vi "main.vi"() -> ()   [LabVIEW 2023]
uses:
  Laser_Ethernet_class/Laser_Ethernet.lvclass
  Laser Ethernet Rack_class/Laser Ethernet Rack.lvclass
  Laser Ethernet Cabinet_class/Laser Ethernet Cabinet.lvclass
  C:/Users/TimBerrier/Code/LabVIEW/Source/APIs/IPG/ipg_tcp/Laser_Ethernet_class/Laser_Ethernet.lvclass
panel:
  in  "Rack?":bool
  in  "address 2":string
  in  "timeout (ms) 2":i32=5000
  in  "remote port or service name 2":u16=5100
  out "Connected 2":bool
  out "error out 2":errorcluster
  out "error out":errorcluster
  out "Connected":bool
  in  "remote port or service name":u16=5100
  in  "timeout (ms)":i32=5000
  in  "address":string
  in  "Name":string
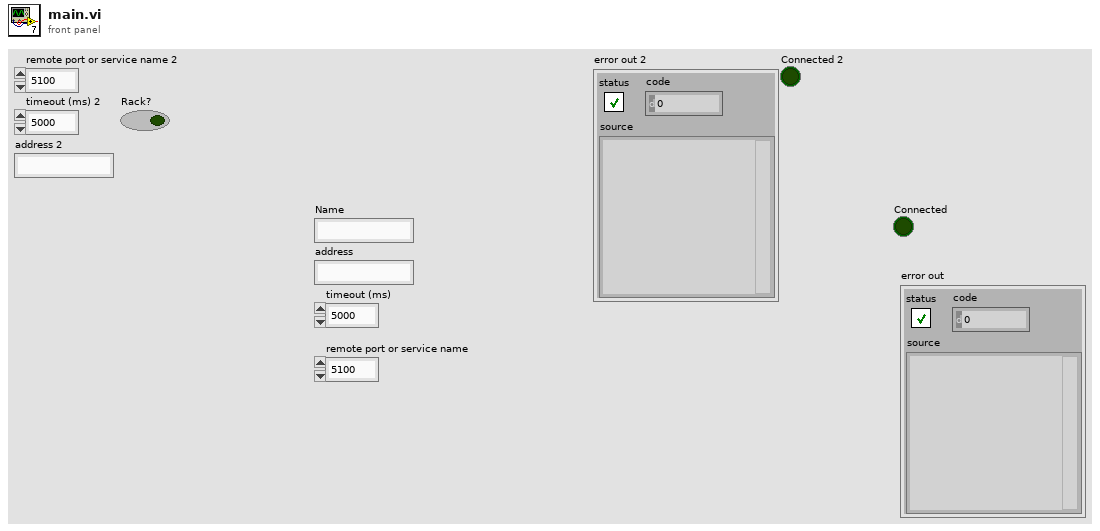
[diagram p1: front panel]
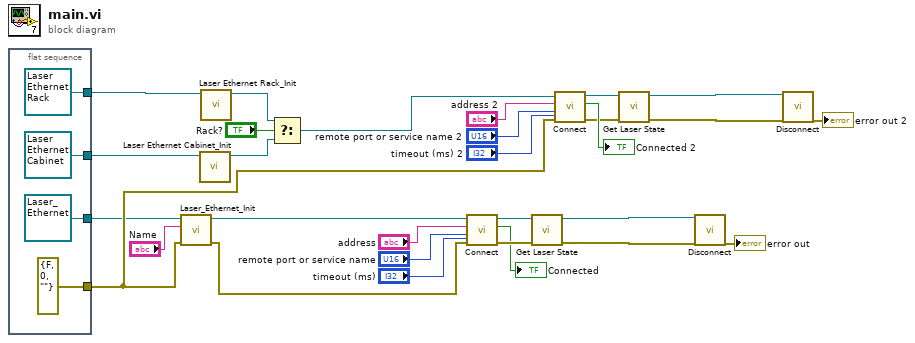
[diagram p0: block diagram]
diagram:
  n1 = flat-sequence {
    tunnel: [refnum<class "Laser_Ethernet.lvclass"> refnum ("object in")] -> w1
    tunnel: [refnum<class "Laser Ethernet Rack.lvclass"> refnum ("object in")] -> w29
    tunnel: [refnum<class "Laser Ethernet Cabinet.lvclass"> refnum ("object in 2")] -> w28
    tunnel: [errorcluster {"status"=FALSE, "code"=0, "source"=""} ("error in (no error)")] -> w2
    frame #0 {
    }
  }
  n2 = call "Laser_Ethernet_Init.vi"("error in (no error)"=w2, "Name"="Name", "object in"=w1) -> ("error out"=w17:errorcluster, "object out"=w26:refnum<class "Laser_Ethernet.lvclass">)  [unwired: 7 in]
  n3 = call "Laser Ethernet Cabinet_Init.vi"("object in"=w28) -> ("object out"=w5:refnum<class "Laser Ethernet Cabinet.lvclass">)  [unwired: 9 in, 1 out]
  n4 = call "Laser Ethernet Rack_Init.vi"("object in"=w29) -> ("object out"=w6:refnum<class "Laser Ethernet Rack.lvclass">)  [unwired: 9 in, 1 out]
  n5 = Select(t=w6, s="Rack?", f=w5) -> (s? t:f=w4:refnum<class "Laser_Ethernet.lvclass">)
  n6 = call-dynamic "Connect.vi"("timeout (ms)"="timeout (ms)", "error in (no error)"=w17, "remote port or service name"="remote port or service name", "address"="address", "object in"=w26) -> ("error out"=w23:errorcluster, "Connected"=→"Connected":bool, "object out"=w24:refnum<class "Laser_Ethernet.lvclass">)  [unwired: 4 in]
  n7 = call-dynamic "Get Laser State.vi"("error in (no error)"=w23, "object in"=w24) -> ("error out"=w21:errorcluster, "object out"=w22:refnum<class "Laser_Ethernet.lvclass">)  [unwired: 7 in, 1 out]
  n8 = call-dynamic "Connect.vi"("timeout (ms)"="timeout (ms) 2", "error in (no error)"=w2, "remote port or service name"="remote port or service name 2", "address"="address 2", "object in"=w4) -> ("error out"=w9:errorcluster, "Connected"=→"Connected 2":bool, "object out"=w8:refnum<class "Laser_Ethernet.lvclass">)  [unwired: 4 in]
  n9 = call-dynamic "Get Laser State.vi"("error in (no error)"=w9, "object in"=w8) -> ("error out"=w11:errorcluster, "object out"=w10:refnum<class "Laser_Ethernet.lvclass">)  [unwired: 7 in, 1 out]
  n10 = call-dynamic "Disconnect.vi"("object in"=w22, "error in (no error)"=w21) -> ("error out"=→"error out":errorcluster)  [unwired: 16 in, 1 out]
  n11 = call-dynamic "Disconnect.vi"("object in"=w10, "error in (no error)"=w11) -> ("error out"=→"error out 2":errorcluster)  [unwired: 16 in, 1 out]
